vi "Compare_values_Modify_Cost_f()-1-2.vi"(4 "[IN] Track Length":u8[](array[numeric]), 5 "[IN] Cost function":i8[](array[numeric]), 6 "[IN] Additions to cost":i8[](array[numeric]), 7 "[IN] Array of displa\ncement differences":dbl[](array[numeric]), 8 "[IN] Statuses of points":i16[](array[numeric]), 9 "[IN] Areas \ndifferences":dbl[](array[numeric]), 10 "[IN] Reverse or not":bool[](array[boolean]), 11 "[IN] Angles betwe\nen displacements":dbl[](array[numeric])) -> (3 "[OUT] Cost function":i8[](array[numeric]))   [LabVIEW 2013]
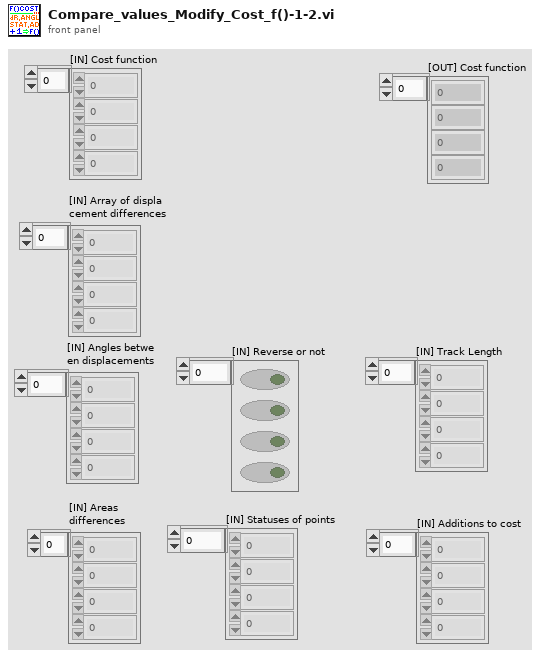
[diagram p1: front panel]
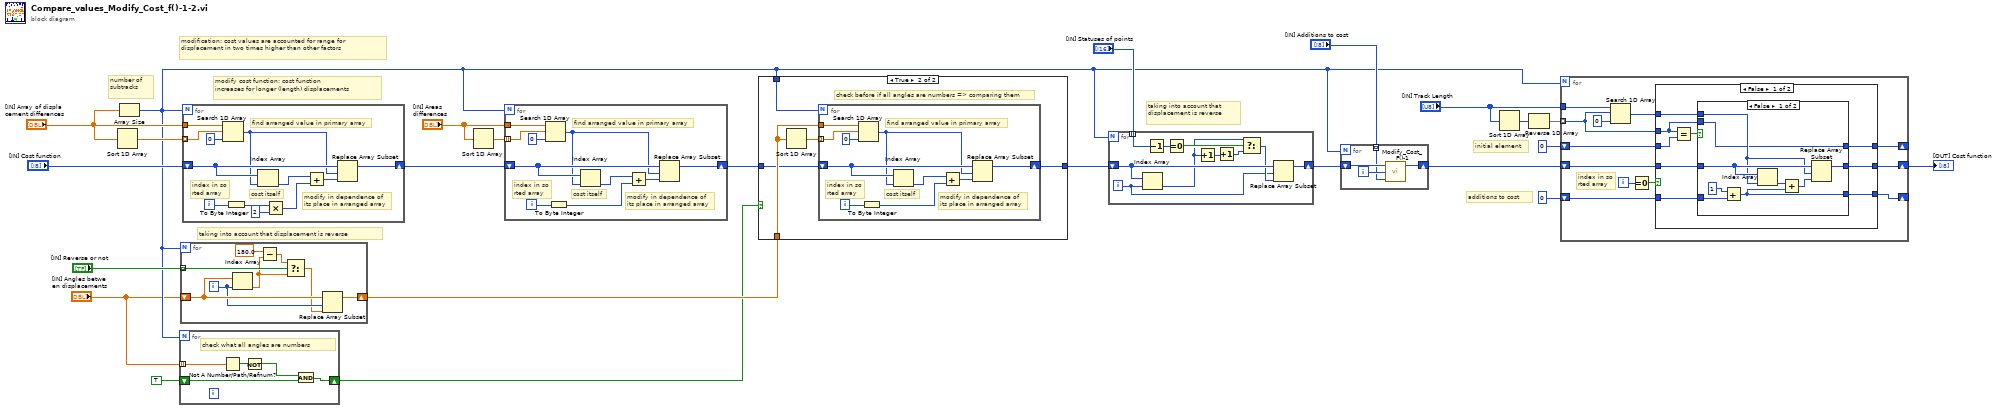
[diagram p0: block diagram]
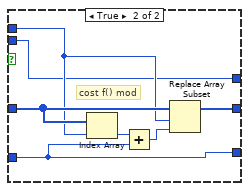
[diagram p3: hidden frame]
diagram:
  # "modification: cost values are accounted for range for \ndisplacement in two times higher than other factors"
  # "additions to cost"
  # "initial element"
  # "taking into account that \ndisplacement is reverse"
  # "taking into account that displacement is reverse"
  # "modify cost function: cost function \nincreases for longer (length) displacements"
  # "number of \nsubtracks"
  n1 = Sort 1D Array(array="[IN] Array of displa\ncement differences") -> (sorted array=w24:dbl[])
  n2 = Array Size(array="[IN] Array of displa\ncement differences") -> (size(s)=w4:i32)
  n3 = for {
    N: w4 -> [_]
    tunnel: "[IN] Angles betwe\nen displacements" -> [w28] mode=indexing
    shift-right: [w25] -> w1
    shift-left: TRUE -> [w29]
    # "check what all angles are numbers"
    n4 = Not A Number/Path/Refnum?(number/path/refnum=w28) -> (NaN/Path/Refnum?=w27:bool)
    n5 = Not(x=w27) -> (.not. x?=w26:bool)
    n6 = And(x=w26, y=w29) -> (x .and. y?=w25:bool)
  }
  n7 = for {
    N: w4 -> [_]
    shift-right: [w30] -> w17
    shift-left: "[IN] Angles betwe\nen displacements" -> [w36]
    tunnel: "[IN] Reverse or not" -> [w37] mode=indexing
    i -> [w32]
    n8 = Index Array(array=w36, index=w32) -> (element=w34:dbl)
    n9 = Subtract(x=180.0, y=w34) -> (x-y=w33:dbl)
    n10 = Select(t=w33, s=w37, f=w34) -> (s? t:f=w31:dbl)
    n11 = Replace Array Subset(array=w36, new element=w31, index=w32) -> (w30:dbl[])
  }
  n12 = for {
    N: w4 -> [_]
    tunnel: w24 -> [w47] mode=indexing
    tunnel: "[IN] Array of displa\ncement differences" -> [w49]
    shift-right: [w41] -> w21
    shift-left: "[IN] Cost function" -> [w46]
    i -> [w42]
    # "modify in dependence of \nits place in arranged array"
    # "find arranged value in primary array"
    # "index in so\nrted array"
    # "cost itself"
    n13 = Search 1D Array(1D array=w49, element=w47, start index (0)=0) -> (index of element=w45:i32)
    n14 = To Byte Integer(number=w42) -> (8bit integer=w40:i8)
    n15 = Index Array(array=w46, index=w45) -> (element=w44:i8)
    n16 = Multiply(x=w40, y=i8 2) -> (x*y=w38:i8)
    n17 = Add(x=w44, y=w38) -> (x+y=w43:i8)
    n18 = Replace Array Subset(array=w46, new element=w43, index=w45) -> (w41:i8[])
  }
  n19 = Sort 1D Array(array="[IN] Areas \ndifferences") -> (sorted array=w19:dbl[])
  n20 = for {
    N: w4 -> [_]
    tunnel: w19 -> [w57] mode=indexing
    tunnel: "[IN] Areas \ndifferences" -> [w59]
    shift-right: [w50] -> w16
    shift-left: w21 -> [w56]
    i -> [w52]
    # "modify in dependence of \nits place in arranged array"
    # "find arranged value in primary array"
    # "index in so\nrted array"
    # "cost itself"
    n21 = Search 1D Array(1D array=w59, element=w57, start index (0)=0) -> (index of element=w55:i32)
    n22 = To Byte Integer(number=w52) -> (8bit integer=w51:i8)
    n23 = Index Array(array=w56, index=w55) -> (element=w54:i8)
    n24 = Add(x=w54, y=w51) -> (x+y=w53:i8)
    n25 = Replace Array Subset(array=w56, new element=w53, index=w55) -> (w50:i8[])
  }
  n26 = case shown="True" w1 {
    tunnel: w17 -> [_ w64]
    tunnel: w16 -> [w60 w63]
    tunnel: [w60 w62] -> w15
    tunnel: w4 -> [_ w61]
    frame False {
    }
    frame True {
      # "check before if all angles are numbers => comparing them"
      n27 = Sort 1D Array(array=w64) -> (sorted array=w65:dbl[])
      n28 = for {
        N: w61 -> [_]
        tunnel: w65 -> [w73] mode=indexing
        tunnel: w64 -> [w75]
        shift-right: [w66] -> w62
        shift-left: w63 -> [w72]
        i -> [w68]
        # "modify in dependence of \nits place in arranged array"
        # "find arranged value in primary array"
        # "index in so\nrted array"
        # "cost itself"
        n29 = Search 1D Array(1D array=w75, element=w73, start index (0)=0) -> (index of element=w71:i32)
        n30 = To Byte Integer(number=w68) -> (8bit integer=w67:i8)
        n31 = Index Array(array=w72, index=w71) -> (element=w70:i8)
        n32 = Add(x=w70, y=w67) -> (x+y=w69:i8)
        n33 = Replace Array Subset(array=w72, new element=w69, index=w71) -> (w66:i8[])
      }
    }
  }
  n34 = for {
    N: w4 -> [_]
    shift-right: [w76] -> w13
    shift-left: w15 -> [w85]
    tunnel: "[IN] Statuses of points" -> [w84] mode=indexing
    i -> [w77]
    n35 = Index Array(array=w85, index=w77) -> (element=w81:i8)
    n36 = Decrement(x=w84) -> (x-1=w83:i16)
    n37 = Equal To 0?(x=w83) -> (x = 0?=w82:bool)
    n38 = Increment(x=w81) -> (x+1=w80:i8)
    n39 = Increment(x=w80) -> (x+1=w79:i8)
    n40 = Select(t=w81, s=w82, f=w79) -> (s? t:f=w78:i8)
    n41 = Replace Array Subset(array=w85, new element=w78, index=w77) -> (w76:i8[])
  }
  n42 = for {
    N: w4 -> [_]
    shift-right: [w86] -> w7
    shift-left: w13 -> [w89]
    tunnel: "[IN] Additions to cost" -> [w87] mode=indexing
    i -> [w88]
    n43 = call "Modify_Cost_F()-1.vi"("[IN] Additions to cost"=w87, "[IN] Current Index"=w88, "[IN] Cost function"=w89) -> ("[OUT] Cost function"=w86:i8[])  [unwired: 2 in]
  }
  n44 = Sort 1D Array(array="[IN] Track Length") -> (sorted array=w11:u8[])
  n45 = Reverse 1D Array(array=w11) -> (reversed array=w10:u8[])
  n46 = for {
    N: w4 -> [_]
    tunnel: w10 -> [w97] mode=indexing
    tunnel: "[IN] Track Length" -> [w101]
    shift-right: [w95] -> w5
    shift-left: w7 -> [w96]
    shift-right: [w94] -> _
    shift-left: u8 0 -> [w93]
    shift-right: [w91] -> _
    shift-left: i8 0 -> [w92]
    i -> [w99]
    # "index in so\nrted array"
    n47 = Search 1D Array(1D array=w101, element=w97, start index (0)=0) -> (index of element=w90:i32)
    n48 = Equal To 0?(x=w99) -> (x = 0?=w98:bool)
    n49 = case shown="False" w98 {
      tunnel: w97 -> [w105 w128]
      tunnel: [w104 w129] -> w95
      tunnel: w96 -> [w108 w129]
      tunnel: [w103 w128] -> w94
      tunnel: w93 -> [w110 _]
      tunnel: [w102 w127] -> w91
      tunnel: w92 -> [w106 w127]
      tunnel: w90 -> [w107 _]
      frame False {
        n50 = Equal?(x=w105, y=w110) -> (x = y?=w109:bool)
        n51 = case shown="False" w109 {
          tunnel: w108 -> [w117 w124]
          tunnel: w107 -> [w114 w121]
          tunnel: w106 -> [w119 w123]
          tunnel: w105 -> [w112 w120]
          tunnel: [w113 w122] -> w104
          tunnel: [w112 w120] -> w103
          tunnel: [w111 w123] -> w102
          frame False {
            n52 = Add(x=i8 1 ("y"), y=w119) -> (x+y=w111:i8)
            n53 = Index Array(array=w117, index=w114) -> (element=w116:i8)
            n54 = Add(x=w116, y=w111) -> (x+y=w115:i8)
            n55 = Replace Array Subset(array=w117, new element=w115, index=w114) -> (w113:i8[])
          }
          frame True {
            # "cost f() mod"
            n56 = Index Array(array=w124, index=w121) -> (element=w125:i8)
            n57 = Add(x=w125, y=w123) -> (x+y=w126:i8)
            n58 = Replace Array Subset(array=w124, new element=w126, index=w121) -> (w122:i8[])
          }
        }
      }
      frame True {
      }
    }
  }
  "[OUT] Cost function" <- w5
